vi "Get Event Timing Windows.vi"(8 "error in (no error)":errorcluster, 10 "Max engine angle":dbl min=0.0 format="%#_f", 11 "Item Ref in":T1 format="%.0x") -> (0 "error out":errorcluster, 2 "Windows":T2[](array[typedef]), 3 "Item Ref out":T1 format="%.0x")   [LabVIEW 2020, in "Engine Simulation Toolkit System Explorer.lvlib"]
uses:
  Engine Simulation Toolkit System Explorer.lvlib
  Event Timing Window.ctl
  <vilib>/NI VeriStand/Custom Device API/Custom Device Item Ref.ctl
  Shared/Properties.vi
  <vilib>/NI VeriStand/Custom Device API/Get Item Property (String Array).vi
  <vilib>/NI VeriStand/Custom Device API/Get Item Property (Double Array).vi
  <vilib>/NI VeriStand/Custom Device API/Custom Device API.lvlib
  Shared/Engine Simulation Toolkit Shared.lvlib
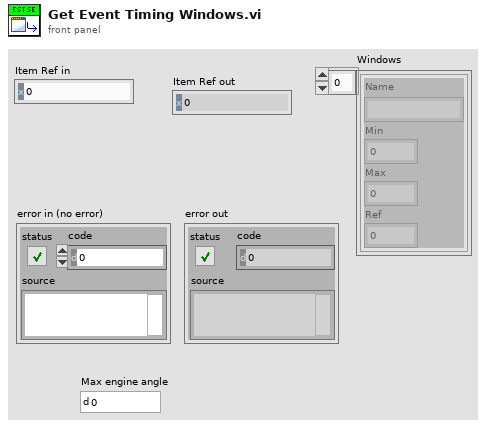
[diagram p1: front panel]
types:
  T1 = typedef "Custom Device API.lvlib/Custom Device Item Ref.ctl" = u64
  T2 = typedef "Engine Simulation Toolkit System Explorer.lvlib/Event Timing Window.ctl" = cluster{"Name":string, "Min":dbl, "Max":dbl, "Ref":dbl}
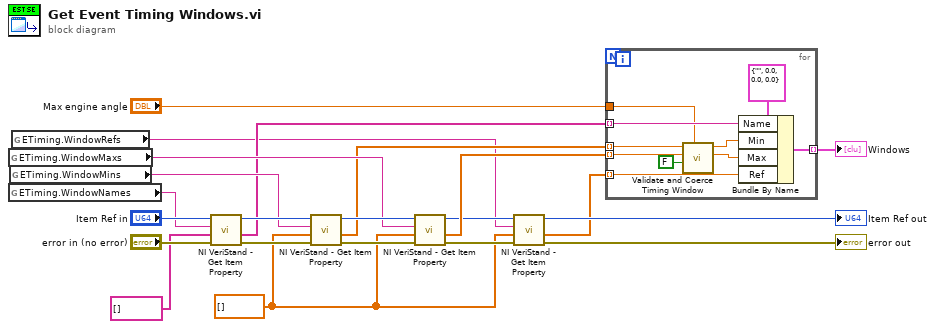
[diagram p0: block diagram]
diagram:
  w3 = dbl[] []
  n1 = global read "Properties.vi" "ETiming.WindowMaxs"() -> (w13:string)
  n2 = global read "Properties.vi" "ETiming.WindowNames"() -> (w20:string)
  n3 = global read "Properties.vi" "ETiming.WindowMins"() -> (w17:string)
  n4 = global read "Properties.vi" "ETiming.WindowRefs"() -> (w2:string)
  n5 = call-poly <vilib>:"NI VeriStand - Get Item Property.vi"("error in (no error)"="error in (no error)", "Default Value"=string[] [], "Property Name"=w20, "Item Ref in"="Item Ref in") -> ("error out"=w18:errorcluster, "Value"=w11:string[], "Item Ref out"=w19:T1)  [unwired: 4 in, 1 out]
  n6 = call-poly <vilib>:"NI VeriStand - Get Item Property.vi"("error in (no error)"=w18, "Default Value"=w3, "Property Name"=w17, "Item Ref in"=w19) -> ("error out"=w15:errorcluster, "Value"=w10:dbl[], "Item Ref out"=w16:T1)  [unwired: 4 in, 1 out]
  n7 = call-poly <vilib>:"NI VeriStand - Get Item Property.vi"("error in (no error)"=w15, "Default Value"=w3, "Property Name"=w13, "Item Ref in"=w16) -> ("error out"=w14:errorcluster, "Value"=w9:dbl[], "Item Ref out"=w5:T1)  [unwired: 4 in, 1 out]
  n8 = call-poly <vilib>:"NI VeriStand - Get Item Property.vi"("error in (no error)"=w14, "Default Value"=w3, "Property Name"=w2, "Item Ref in"=w5) -> ("error out"=→"error out":errorcluster, "Value"=w1:dbl[], "Item Ref out"=→"Item Ref out":T1)  [unwired: 4 in, 1 out]
  n9 = for {
    tunnel: w11 -> [w31] mode=indexing
    tunnel: w10 -> [w27] mode=indexing
    tunnel: w9 -> [w26] mode=indexing
    tunnel: [w30] -> w8 mode=indexing
    tunnel: "Max engine angle" -> [w28]
    tunnel: w1 -> [w23] mode=indexing
    n10 = call "Validate and Coerce Timing Window.vi"("Max engine angle"=w28, "Min changed last"=FALSE, "Max"=w26, "Min"=w27) -> ("Coerced maximum"=w25:dbl, "Coerced minimum"=w24:dbl)  [unwired: 6 in]
    n11 = Bundle By Name(cluster=T2 {"Name"="", "Min"=0.0, "Max"=0.0, "Ref"=0.0} ("Window"), "Name"=w31, "Min"=w24, "Max"=w25, "Ref"=w23) -> (w30:T2)
  }
  "Windows" <- w8
